vi "TimerEngine.Template.vi"(8 "error in (no error)":errorcluster) -> (0 "error out":errorcluster)   [LabVIEW 2017, in "TimerEngine.lvlib" / "TimerEngine.lvclass"]
uses:
  TimerEngine.lvclass
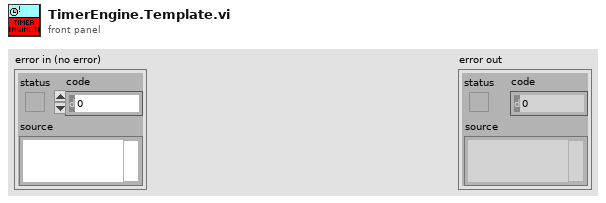
[diagram p1: front panel]
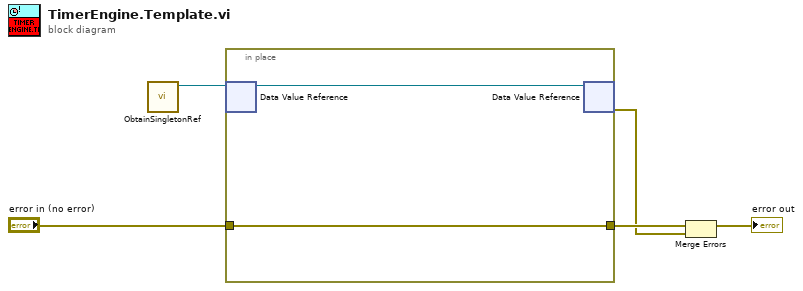
[diagram p0: block diagram]
diagram:
  n1 = call "ObtainSingletonRef.vi"() -> ("data value reference"=w5:refnum<data-value>)  [unwired: 10 in, 1 out]
  n2 = in-place {
    in-place-border: [w6] -> w4
    in-place-border: "error in (no error)" -> [w6]
    n3 = in-place-dvr #1(w5) -> (w7:refnum<class "TimerEngine.lvclass">)  [unwired: 1 out]
    n4 = in-place-dvr #1(w7) -> (w1:errorcluster)  [unwired: 1 out]
  }
  n5 = Merge Errors(w4, w1) -> (→"error out":errorcluster)
